vi "cDAQ_VI_Leo_Modified_1.vi"() -> ()   [LabVIEW 2022 SP3]
uses:
  <vilib>/Utility/error.llb/DialogType.ctl
  <vilib>/DAQmx/read.llb/DAQmx Read (Analog 1D Wfm NChan NSamp).vi
  <vilib>/Analysis/baseanly.llb/Mean (DBL).vi
  <vilib>/DAQmx/create/channels.llb/DAQmx Create Channel (AI-Voltage-Basic).vi
  <vilib>/DAQmx/create/channels.llb/DAQmx Create Channel (AI-Force-Bridge-Two-Point-Linear).vi
  <vilib>/DAQmx/configure/timing.llb/DAQmx Timing (Sample Clock).vi
  STOP_GLOBAL.vi
  <vilib>/DAQmx/miscellaneous.llb/DAQmx Fill In Error Info.vi
  <vilib>/Analysis/NI_AALBase.lvlib
panel:
  out "Chamber Pressure PSI 2":dynamicdata(graph)
  out "Thrust lb 2":dynamicdata(graph)
  in  "Enable 2":bool=TRUE caption="Enable"
  in  "Enable":bool=TRUE
  out "date string":string
  out "Thrust":dbl[](graph)
  out "Numeric 2":i32
  in  "Types of Testing":enum32{"Test Firing", "Cold Flow Rig"}(tab)
  out "Saving Data":bool
  out "Filename Out":path
  in  "Data Collection Folder":path
  in  "File Name Voltage 9219":string
  in  "File Name Thrust":string
  in  "File Name Temp":string
  in  "File Format":string
  out "Saving Data":bool
  out "Filename Out 5":path caption="Filename Out"
  in  "Filename 5":path=path "C:/1. Rocket Research Project/CollectedData/Calibrations/Thrust_Testing_7.lvm" caption="Filename"
  # "DATA LOGGING INFORMATION"
  # "ANALOG VOLTAGE OUTPUT"
  # "RESULTS"
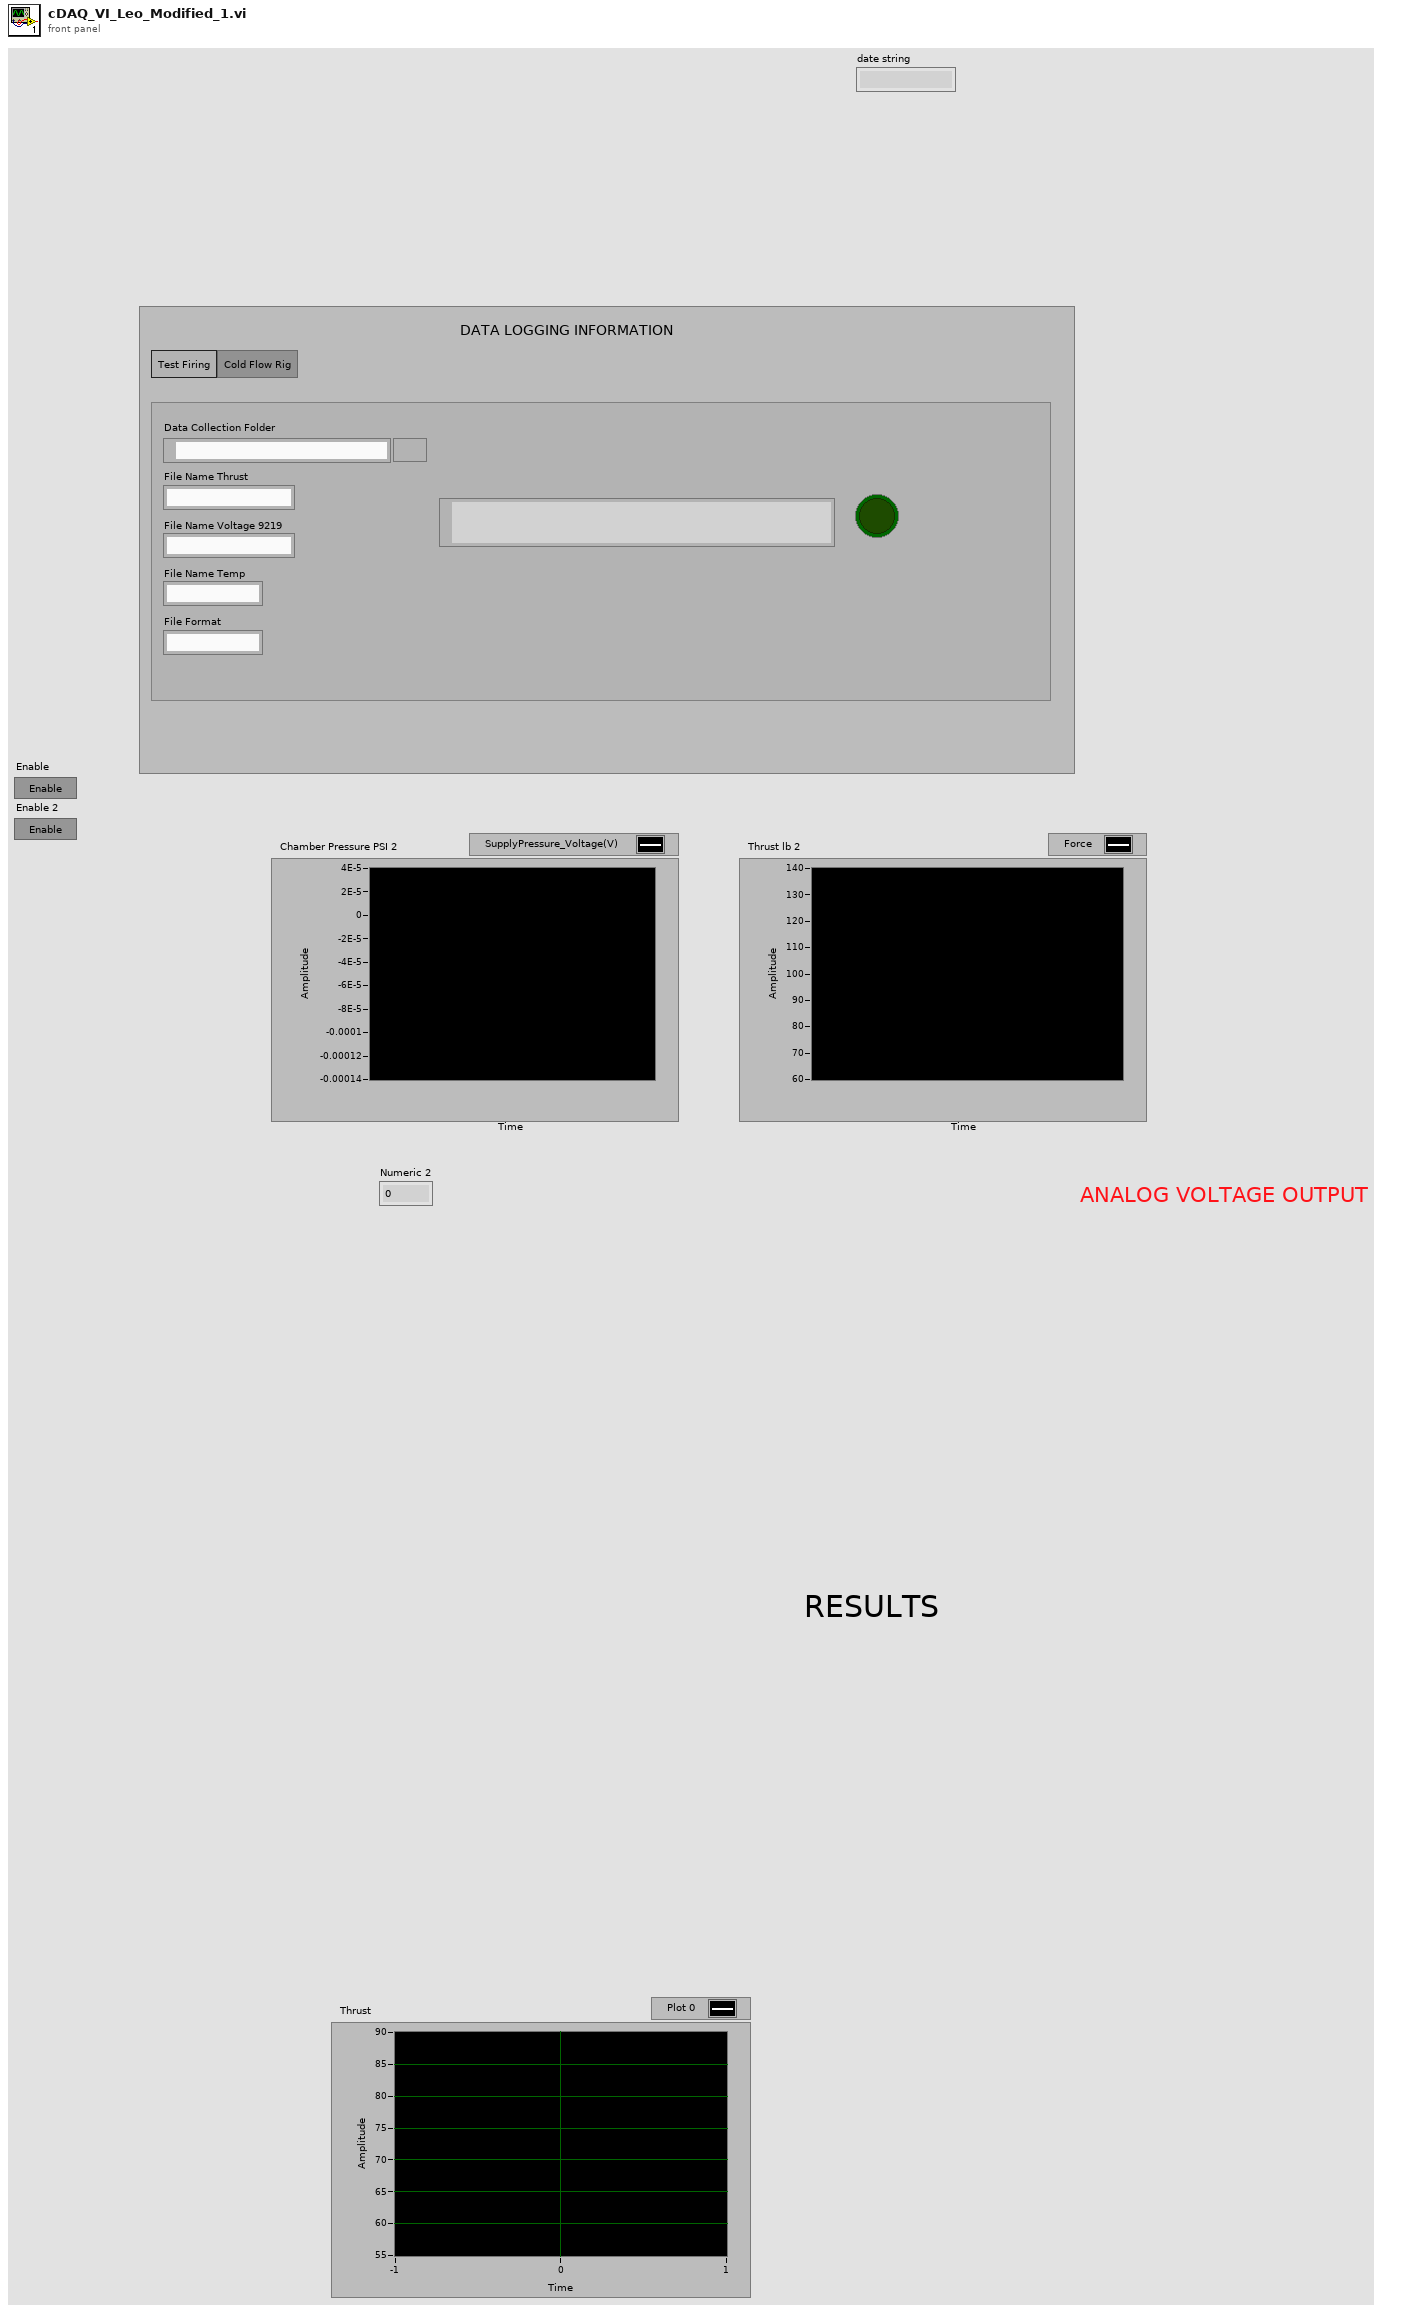
[diagram p1: front panel]
types:
  T1 = typedef "DialogType.ctl" = u16
  T2 = cluster{"bridge configuration":i32, "voltage excitation source":i32, "voltage excitation value":dbl, "nominal bridge resistance":dbl}
  T3 = cluster{"first electrical value":dbl, "second electrical value":dbl, "electrical units":i32, "first physical value":dbl, "second physical value":dbl, "physical units":i32}
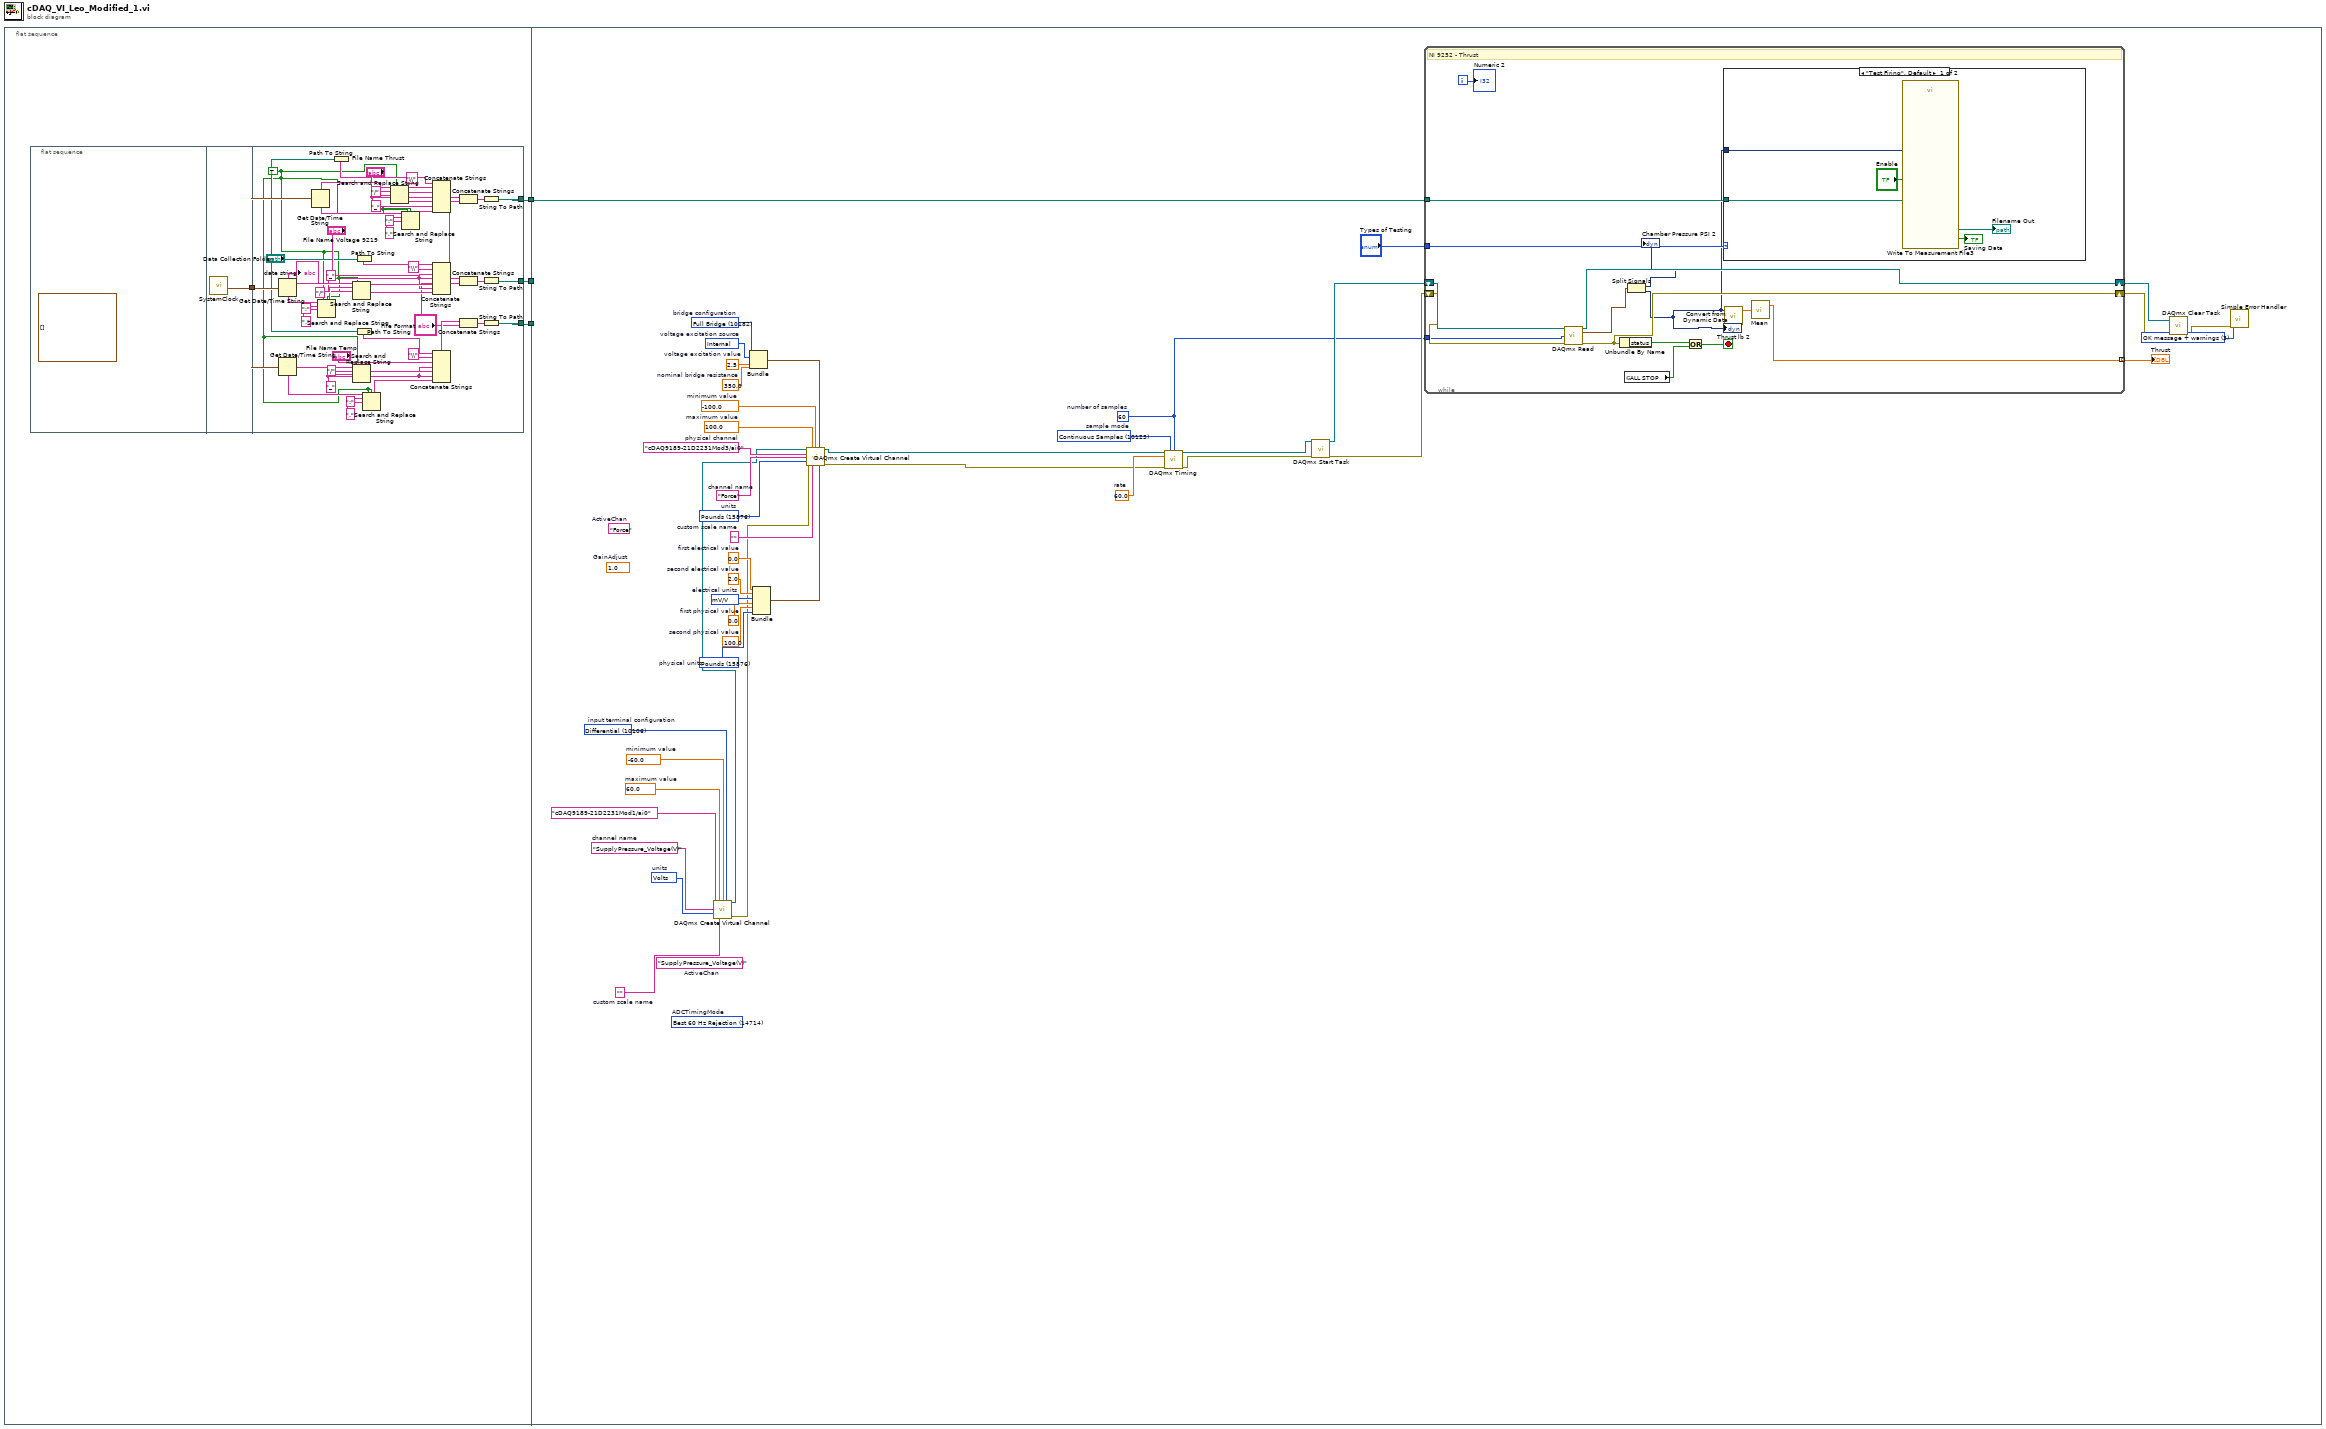
[diagram p0: block diagram]
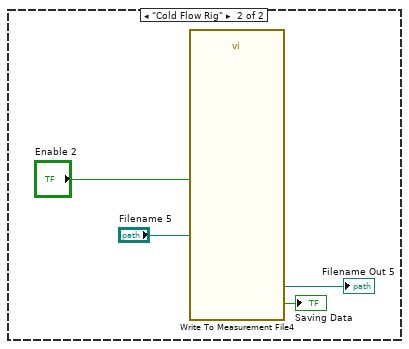
[diagram p2: hidden frame]
diagram:
  n1 = flat-sequence {
    tunnel: [w6] -> w3
    tunnel: [w5] -> w2
    tunnel: [w4] -> w1
    tunnel: w3 -> [_]
    tunnel: w2 -> [_]
    tunnel: w1 -> [w95]
    frame #0 {
      n2 = flat-sequence {
        tunnel: [w8] -> w7
        tunnel: w7 -> [w16]
        tunnel: [w41] -> w6
        tunnel: [w14] -> w5
        tunnel: [w13] -> w4
        frame #0 {
          (unwired) waveform(dbl)[] []
        }
        frame #1 {
          n3 = call "SystemClock.vi"() -> ("LabVIEW Time Stamp"=w8:timestamp)  [unwired: 10 in, 1 out]
        }
        frame #2 {
          w9 = TRUE ("replace all? (F)")
          w24 = "_" ("string")
          w32 = "_" ("string")
          w45 = "_" ("string")
          n4 = Get Date/Time String(seconds (now)=w16) -> (date string=w38:string, time string=w35:string)  [unwired: 2 in]
          "date string" <- w38
          n5 = Get Date/Time String(seconds (now)=w16) -> (date string=w51:string, time string=w48:string)  [unwired: 2 in]
          n6 = Get Date/Time String(seconds (now)=w16) -> (date string=w18:string, time string=w21:string)  [unwired: 2 in]
          n7 = Search and Replace String(replace all?=w9, case sensitive?=w9, input string=w35, search string=":", replace string="." ("replace string (\"\")")) -> (result string=w31:string)  [unwired: 3 in, 3 out]
          n8 = Path To String(path="Data Collection Folder") -> (string=w11:string)
          n9 = Search and Replace String(replace all?=w9, input string=w38, search string="/", replace string=w32) -> (result string=w36:string)  [unwired: 4 in, 3 out]
          n10 = Search and Replace String(replace all?=w9, input string=w51, search string="/", replace string=w45) -> (result string=w49:string)  [unwired: 4 in, 3 out]
          n11 = Path To String(path="Data Collection Folder") -> (string=w28:string)
          n12 = Path To String(path="Data Collection Folder") -> (string=w53:string)
          n13 = Search and Replace String(replace all?=w9, case sensitive?=w9, input string=w48, search string=":", replace string="." ("replace string (\"\")")) -> (result string=w44:string)  [unwired: 3 in, 3 out]
          n14 = Search and Replace String(replace all?=w9, input string=w18, search string="/", replace string=w24) -> (result string=w20:string)  [unwired: 4 in, 3 out]
          n15 = Search and Replace String(replace all?=w9, case sensitive?=w9, input string=w21, search string=":", replace string="." ("replace string (\"\")")) -> (result string=w25:string)  [unwired: 3 in, 3 out]
          n16 = Concatenate Strings(w11, "\\" ("string"), "File Name Thrust", w24, w20, w24, w25) -> (w26:string)
          n17 = Concatenate Strings(w28, "\\" ("string"), "File Name Voltage 9219", w32, w36, w32, w31) -> (w30:string)
          n18 = Concatenate Strings(w53, "\\" ("string"), "File Name Temp", w45, w49, w45, w44) -> (w43:string)
          n19 = Concatenate Strings(w26, "File Format") -> (w27:string)
          n20 = Concatenate Strings(w30, "File Format") -> (w29:string)
          n21 = Concatenate Strings(w43, "File Format") -> (w42:string)
          n22 = String To Path(string=w27) -> (path=w13:path)
          n23 = String To Path(string=w29) -> (path=w14:path)
          n24 = String To Path(string=w42) -> (path=w41:path)
        }
      }
    }
    frame #1 {
      w56 = T1 3 items=["no dialog", "OK message", "continue or stop message", "OK message + warnings", "continue/stop + warnings"] ("type of dialog (OK msg:1)")
      (unwired) 14714 items=["High Resolution"=10195, "High Speed"=14712, "Best 50 Hz Rejection"=14713, "Best 60 Hz Rejection"=14714]  # ADCTimingMode
      (unwired) "SupplyPressure_Voltage(V)"  # ActiveChan
      w69 = 10106 items=["default"=-1, "RSE"=10083, "NRSE"=10078, "Differential"=10106, "Pseudodifferential"=12529]  # input terminal configuration
      w70 = 10348 items=["Volts"=10348, "From Custom Scale"=10065]  # units
      w71 = "SupplyPressure_Voltage(V)"  # channel name
      w72 = ""  # custom scale name
      w73 = -60.0  # minimum value
      w74 = 60.0  # maximum value
      w75 = 10123 items=["Finite Samples"=10178, "Continuous Samples"=10123, "Hardware Timed Single Point"=12522]  # sample mode
      w76 = 60.0  # rate
      w55 = 60  # number of samples
      (unwired) 1.0  # GainAdjust
      (unwired) "Force"  # ActiveChan
      w77 = 15876 items=["Newtons"=15875, "Pounds"=15876, "kgf"=15877]  # physical units
      w83 = 0.0  # first electrical value
      w82 = 2.0  # second electrical value
      w81 = 15897 items=["V/V"=15896, "mV/V"=15897]  # electrical units
      w80 = 0.0  # first physical value
      w79 = 100.0  # second physical value
      w85 = 350.0  # nominal bridge resistance
      w86 = 2.5  # voltage excitation value
      w87 = 10200 items=["Internal"=10200, "External"=10167]  # voltage excitation source
      w88 = 10182 items=["Full Bridge"=10182, "Half Bridge"=10187, "Quarter Bridge"=10270]  # bridge configuration
      w89 = 15876 items=["Newtons"=15875, "Pounds"=15876, "kgf"=15877, "From Custom Scale"=10065]  # units
      w90 = "Force"  # channel name
      w91 = ""  # custom scale name
      w92 = -100.0  # minimum value
      w93 = 100.0  # maximum value
      w94 = "cDAQ9189-21D2231Mod3/ai0"  # physical channel
      n25 = call-poly <vilib>:"DAQmx Create Virtual Channel.vi"("maximum value"=w74, "minimum value"=w73, "input terminal configuration"=w69, "physical channels"=tag "cDAQ9189-21D2231Mod1/ai0", "name to assign"=w71, "units"=w70, "custom scale name"=w72) -> ("task out"=w67:refnum<k21>, "error out"=w64:errorcluster)  [unwired: 7 in]
      n26 = Bundle("bridge configuration"=w88, "voltage excitation source"=w87, "voltage excitation value"=w86, "nominal bridge resistance"=w85) -> (w84:T2)  [unwired: 1 in]
      n27 = Bundle("first electrical value"=w83, "second electrical value"=w82, "electrical units"=w81, "first physical value"=w80, "second physical value"=w79, "physical units"=w77) -> (w78:T3)  [unwired: 1 in]
      n28 = call-poly <vilib>:"DAQmx Create Virtual Channel.vi"("task in"=w67, "maximum value"=w93, "minimum value"=w92, "bridge information"=w84, "physical channels"=w94, "name to assign"=w90, "units"=w89, "error in"=w64, "custom scale name"=w91, "scaling information"=w78) -> ("task out"=w66:refnum<k21>, "error out"=w65:errorcluster)  [unwired: 4 in]
      n29 = call-poly <vilib>:"DAQmx Timing.vi"("task/channels in"=w66, "sample mode"=w75, "samples per channel"=w55, "rate"=w76, "error in"=w65) -> ("task out"=w63:refnum<k21>, "error out"=w62:errorcluster)  [unwired: 9 in]
      n30 = call <vilib>:"DAQmx Start Task.vi"("task/channels in"=w63, "error in"=w62) -> ("task out"=w61:refnum<k21>, "error out"=w60:errorcluster)  [unwired: 12 in]
      n31 = while {
        tunnel: "Types of Testing" -> [w112]
        tunnel: [w110] -> w97 mode=indexing
        tunnel: w95 -> [w106]
        shift-right: [w103] -> w59
        shift-left: w61 -> [w104]
        shift-right: [w101] -> w58
        shift-left: w60 -> [w102]
        tunnel: w55 -> [w98]
        i -> [w113]
        stop <- w107 stop-if-true
        # "NI 9252 - Thrust"
        n32 = call-poly <vilib>:"DAQmx Read.vi"("task/channels in"=w104, "number of samples per channel"=w98, "error in"=w102) -> ("task out"=w103:refnum<k21>, "data"=w105:waveform(dbl)[], "error out"=w101:errorcluster)  [unwired: 10 in]
        n33 = Unbundle By Name(w101) -> ("status"=w109:bool)
        n34 = global read "STOP_GLOBAL.vi" "ALL STOP"() -> (w108:bool)
        n35 = Split Signals(w105) -> (→"Chamber Pressure PSI 2":dynamicdata, w100:dynamicdata)  [unwired: 2 in]
        "Thrust lb 2" <- w100
        n36 = Or(x=w109, y=w108) -> (x .or. y?=w107:bool)
        n37 = case shown="\"Test Firing\", Default" w112 {
          tunnel: w100 -> [w116 _]
          tunnel: w106 -> [w115 _]
          frame "Test Firing", Default {
            n38 = call "Write To Measurement File3"("Signals"=w116, "Enable"="Enable", "Filename"=w115) -> ("Filename Out"=→"Filename Out":path, "Saving Data"=→"Saving Data":bool)  [unwired: 14 in, 1 out]
          }
          frame "Cold Flow Rig" {
            n39 = call "Write To Measurement File4"("Enable"="Enable 2", "Filename"="Filename 5") -> ("Filename Out"=→"Filename Out 5":path, "Saving Data"=→"Saving Data":bool)  [unwired: 15 in, 1 out]
          }
        }
        n40 = call "Convert from Dynamic Data"("Dynamic Data Type"=w100) -> ("Array"=w111:dbl[])  [unwired: 3 in]
        n41 = call-poly <vilib>:"Mean.vi"("X"=w111) -> ("mean"=w110:dbl)  [unwired: 1 out]
        "Numeric 2" <- w113
      }
      "Thrust" <- w97
      n42 = call <vilib>:"DAQmx Clear Task.vi"("task in"=w59, "error in"=w58) -> ("error out"=w57:errorcluster)  [unwired: 13 in]
      n43 = call <vilib>:"Simple Error Handler.vi"("type of dialog (OK msg:1)"=w56, "error in (no error)"=w57) -> ()  [unwired: 3 in, 5 out]
    }
  }
